vi "Teleop.vi"(10 "Match Info":T4={"Autonomous Elapsed Seconds"=0.0, "TeleOp Elapsed Seconds"=60.541, "Disabled Elapsed Seconds"=98.983, "Visited Autonomous"=FALSE, "Visited TeleOp"=TRUE, "Visited Disabled"=TRUE, "Autonomous Settings"={"Autonomous Style"=enum."Independent", "VI Refnum"=refnum}}, 11 "Call Context":T5=enum."Stop") -> ()   [LabVIEW 2016]
doc: "This VI is called for each TeleOp packet received from the DS where the robot is not disabled. It is often used to read from the joysticks and update I/O or to update setpoints for timed control loops. It should complete and return within 20 milliseconds or it may miss DS packets."
uses:
  <vilib>/Rock Robotics/WPI/DriverStation/WPI_DriverStationDerivedRobotMode.ctl
  <vilib>/Rock Robotics/WPI/DriverStation/WPI_DriverStationMatch Info.ctl
  <vilib>/Rock Robotics/WPI/Solenoid/WPI_SolenoidValue.ctl
  <vilib>/Rock Robotics/WPI/Utilities/WPI_GetSetVariantRefNum.vi
  <vilib>/Rock Robotics/Network Tables/NT Write Boolean Array.vi
  <vilib>/Rock Robotics/Network Tables/NT Write Numeric Array.vi
  <vilib>/Rock Robotics/Network Tables/NT Read Boolean.vi
  <vilib>/Rock Robotics/Network Tables/NT Read Number.vi
  <vilib>/Rock Robotics/WPI/Solenoid/WPI_SolenoidSetEnum.vi
  <vilib>/addons/control/pid/pid.llb/PID (DBL).vi
  <vilib>/Rock Robotics/WPI/RobotDrive/WPI_RobotDriveMecanumDrive_Cartesian.vi
  <vilib>/Rock Robotics/Network Tables/NT Write Number.vi
  <vilib>/addons/control/pid/NI_PID_pid.lvlib
panel:
  in  "climberpower":dbl(slide)=0.3 scale=0.0..1.0
  in  "deadband thing":dbl=0.13
  in  "Strafe":dbl(slide)=0.5 caption="Strafe Scale" scale=0.0..1.0
  in  "Deadband":dbl(slide) scale=-1.0..1.0
  out "useless data point LOL":dbl=-122.49
  out "derivative time (Td, min)":dbl
  out "integral time (Ti, min)":dbl=0.01
  out "proportional gain (Kc)":dbl=1.0
  out "Yaw":dbl=-122.49
  out "Data":T1(graph)={"setpoint"=0.0, "Yaw"=-122.49, "dt out (s)"=0.02300000109244138}
  in  "setpoint":dbl(slide) scale=-50.0..50.0
  in  "PID gains":T2={"proportional gain (Kc)"=1.0, "integral time (Ti, min)"=0.01, "derivative time (Td, min)"=0.0} {"derivative time (Td, min)" scale=0.0..0.05; "integral time (Ti, min)" scale=0.0..0.00243; "proportional gain (Kc)" scale=0.0..0.284195}
  out "YRPHfH":T3={"Yaw"=-122.49, "Roll"=8.03, "Pitch"=-3.82, "Heading"=0.0, "Fused Heading"=237.5}
  out "Sample Slider 0":dbl(slide) scale=0.0..5.0
  out "Sample Boolean 1":bool
  out "Sample Boolean 0":bool
  # "z check should be about 3-5 (in degrees)"
  # "do not mess with PID gain values"
  # "do not mess with PID gain values"
  # "do not mess with PID gain values"
  # "do not mess with PID gain values"
  # "do not mess with PID gain values"
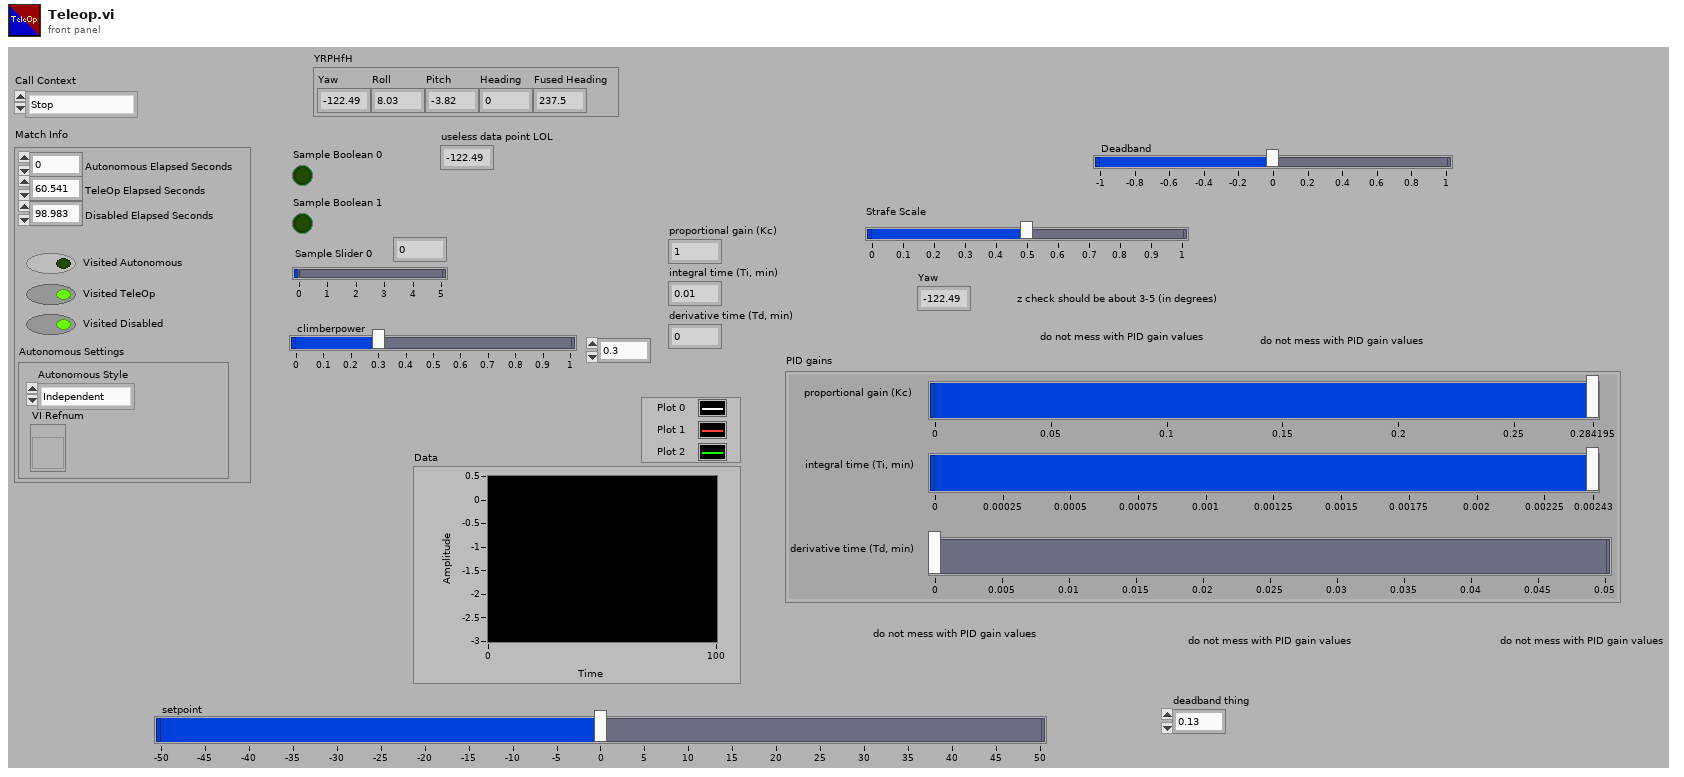
[diagram p1: front panel]
types:
  T1 = cluster{"setpoint":dbl, "Yaw":dbl, "dt out (s)":dbl}
  T2 = cluster{"proportional gain (Kc)":dbl, "integral time (Ti, min)":dbl, "derivative time (Td, min)":dbl}
  T3 = cluster{"Yaw":dbl, "Roll":dbl, "Pitch":dbl, "Heading":dbl, "Fused Heading":dbl}
  T4 = typedef "WPI_DriverStationMatch Info.ctl" = cluster{"Autonomous Elapsed Seconds":dbl, "TeleOp Elapsed Seconds":dbl, "Disabled Elapsed Seconds":dbl, "Visited Autonomous":bool, "Visited TeleOp":bool, "Visited Disabled":bool, "Autonomous Settings":cluster{"Autonomous Style":enum16{"Iterative", "Independent"}, "VI Refnum":refnum<vi>}}
  T5 = typedef "WPI_DriverStationDerivedRobotMode.ctl" = enum16{"Init", "Execute", "Stop"}
  T6 = typedef "WPI_SolenoidValue.ctl" = enum16{"Off", "On", "Forward", "Reverse"}
  T7 = typedef "WPI_JoystickDevRef.ctl" = cluster{"Device":T8}
  T8 = typedef "WPI_JoystickDeviceEnum.ctl" = enum16{"USB 0", "USB 1", "USB 2", "USB 3", "USB 4", "USB 5"}
  T9 = typedef "WPI_MotorControlDeviceRef.ctl" = cluster{"DeviceStatus":errorcluster, "Type":T10, "PWM":cluster{"PWM Channel":T11, "DeadBand":T12}, "CAN":cluster{"Device Number":u8, "SetOutput VI Ref":variant, "GetOutput VI Ref":variant, "Enable VI Ref":variant, "Disable VI Ref":variant, "Data":variant}, "Invert":bool}
  T10 = typedef "WPI_MotorControlType.ctl" = enum16{"PWM", "CAN"}
  T11 = typedef "FPGA_DIOPWMChannel.ctl" = enum8{"PWM 0", "PWM 1", "PWM 2", "PWM 3", "PWM 4", "PWM 5", "PWM 6", "PWM 7", "PWM 8", "PWM 9", "PWM MXP 0", "PWM MXP 1", "PWM MXP 2", "PWM MXP 3", "PWM MXP 4", "PWM MXP 5", "PWM MXP 6", "PWM MXP 7", "PWM MXP 8", "PWM MXP 9", "Invalid"}
  T12 = typedef "WPI_PWMDeadband.ctl" = cluster{"Name":string, "maxPositivePwm":i32, "minPositivePwm":i32, "centerPwm":i32, "maxNegativePwm":i32, "minNegativePwm":i32, "angularRange":u16}
  T13 = typedef "WPI_SolenoidDevRef.ctl" = cluster{"DevStatus":errorcluster, "Pneumatics Control Module":u8, "Forward Solenoid Channel":T14, "Reverse Solenoid Channel":T14}
  T14 = typedef "WPI_SolenoidChannel.ctl" = enum8{"Solenoid 0", "Solenoid 1", "Solenoid 2", "Solenoid 3", "Solenoid 4", "Solenoid 5", "Solenoid 6", "Solenoid 7", "Invalid"}
  T15 = typedef "WPI_RobotDriveDevRef.ctl" = cluster{"DevStatus":errorcluster, "Motors[]":T9[], "Square Inputs":bool, "Max Output":dbl}
  T16 = typedef "WPI_CompressorDevRef.ctl" = cluster{"DevStatus":errorcluster, "Pneumatics Control Module":u8}
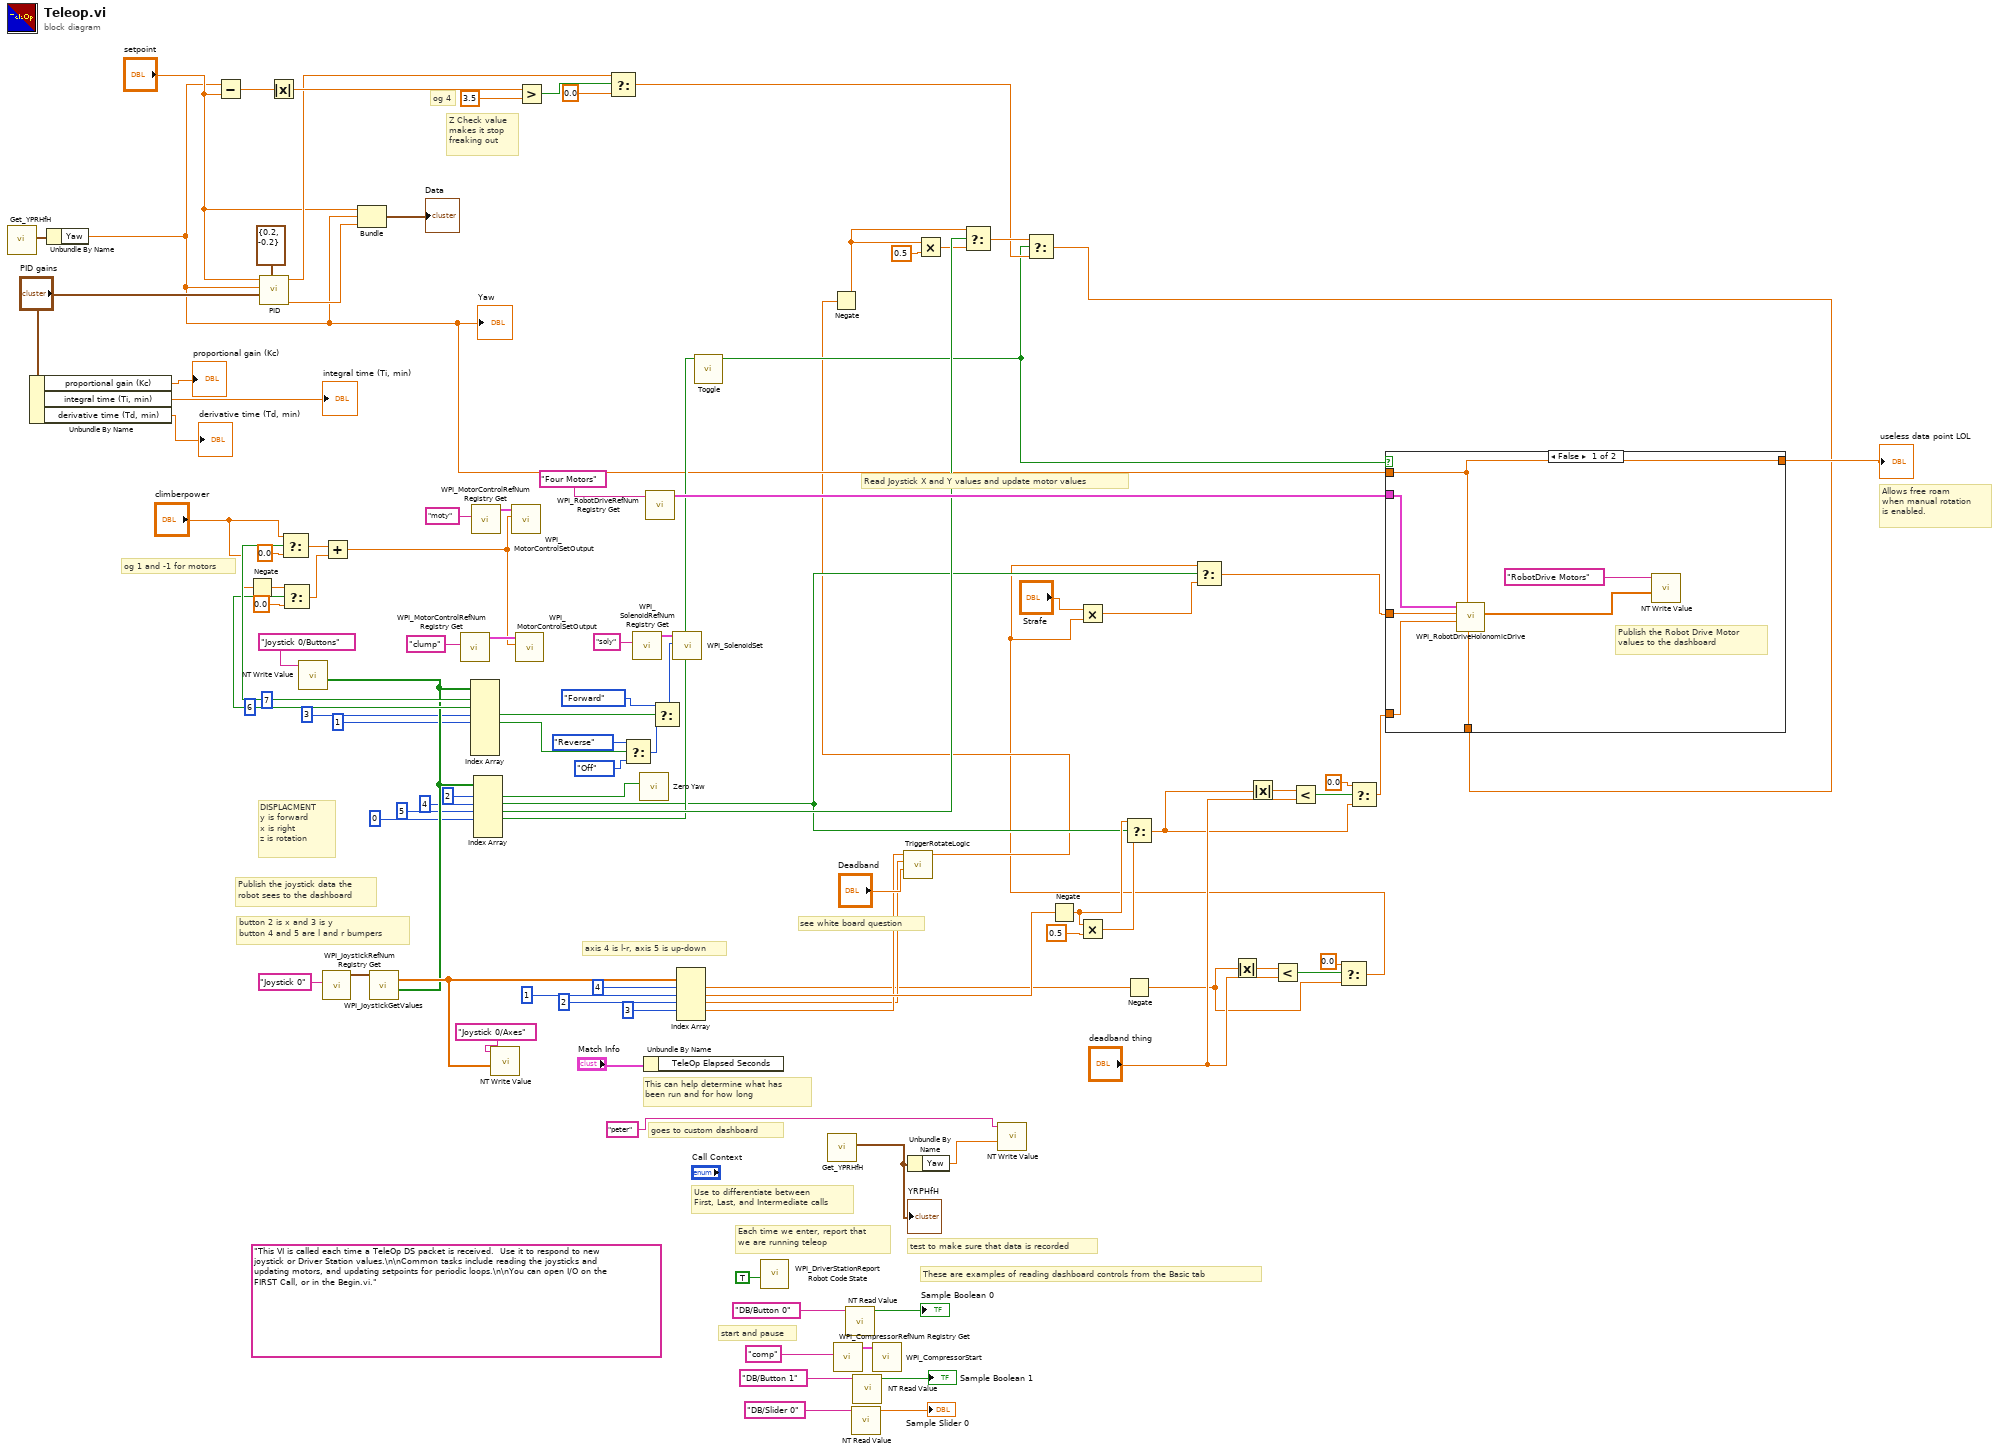
[diagram p0: block diagram]
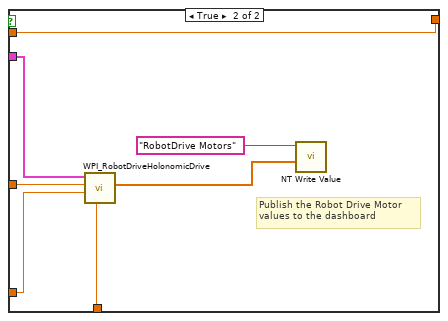
[diagram p2: hidden frame]
diagram:
  (unwired) "This VI is called each time a TeleOp DS packet is received.  Use it to respond to new joystick or Driver Station values.\n\nCommon tasks include reading the joysticks and updating motors, and updating setpoints for periodic loops.\n\nYou can open I/O on the FIRST Call, or in the Begin.vi."
  # "see white board question"
  # "axis 4 is l-r, axis 5 is up-down"
  # "og 1 and -1 for motors"
  # "og 4"
  # "Allows free roam\nwhen manual rotation\nis enabled."
  # "Z Check value\nmakes it stop\nfreaking out"
  # "start and pause"
  # "goes to custom dashboard"
  # "button 2 is x and 3 is y\nbutton 4 and 5 are l and r bumpers"
  # "DISPLACMENT\ny is forward\nx is right\nz is rotation"
  # "test to make sure that data is recorded"
  # "These are examples of reading dashboard controls from the Basic tab"
  # "Publish the joystick data the\nrobot sees to the dashboard"
  # "Each time we enter, report that\nwe are running teleop"
  # "Use to differentiate between\nFirst, Last, and Intermediate calls"
  # "This can help determine what has\nbeen run and for how long"
  # "Read Joystick X and Y values and update motor values"
  n1 = call <vilib>:"Get_YPRHfH.vi"() -> ("YRPHfH"=w49:T3)  [unwired: 11 in]
  n2 = Unbundle By Name("PID gains") -> ("proportional gain (Kc)"=→"proportional gain (Kc)":dbl, "integral time (Ti, min)"=→"integral time (Ti, min)":dbl, "derivative time (Td, min)"=→"derivative time (Td, min)":dbl)
  n3 = Unbundle By Name(w49) -> ("Yaw"=w15:dbl)
  "Yaw" <- w15
  n4 = Subtract(x=w15, y="setpoint") -> (x-y=w53:dbl)
  n5 = Negate(x="climberpower") -> (-x=w1:dbl)
  n6 = call-poly <vilib>:"PID.vi"("output range"=cluster{"output high":dbl, "output low":dbl} {"output high"=0.2, "output low"=-0.2}, "PID gains"="PID gains", "process variable"=w15, "setpoint"="setpoint") -> ("dt out (s)"=w46:dbl, "output"=w45:dbl)  [unwired: 6 in]
  n7 = Absolute Value(x=w53) -> (abs(x)=w54:dbl)
  n8 = call <vilib>:"WPI_JoystickRefNum Registry Get.vi"("refnum name"="Joystick 0") -> ("JoystickDevRef"=w102:T7)  [unwired: 1 in, 9 out]
  n9 = Bundle("setpoint"="setpoint", "Yaw"=w15, "dt out (s)"=w46) -> (→"Data":T1)  [unwired: 1 in]
  n10 = call <vilib>:"WPI_JoystickGetValues.vi"("JoystickDevRef"=w102) -> ("Buttons"=w70:bool[], "Axes"=w99:dbl[])  [unwired: 6 in, 3 out]
  n11 = call-poly <vilib>:"NT Write Value.vi"("Boolean Array"=w70, "Name"="Joystick 0/Buttons") -> ()  [unwired: 9 in, 1 out]
  n12 = call <vilib>:"WPI_MotorControlRefNum Registry Get.vi"("refnum name"="clump") -> ("MotorControlDevRef"=w62:T9)  [unwired: 9 in, 1 out]
  n13 = Index Array(array=w70, index #1=7 ("index"), index #2=6 ("index"), index #3=3 ("index"), index #4=1 ("index")) -> (element #1=w87:bool, element #2=w86:bool, element #3=w23:bool, element #4=w21:bool)  [unwired: 4 in, 4 out]
  n14 = Select(t="climberpower", s=w87, f=0.0) -> (s? t:f=w83:dbl)
  n15 = Select(t=w1, s=w86, f=0.0) -> (s? t:f=w82:dbl)
  n16 = Add(x=w83, y=w82) -> (x+y=w61:dbl)
  n17 = call <vilib>:"WPI_MotorControlRefNum Registry Get.vi"("refnum name"="moty") -> ("MotorControlDevRef"=w88:T9)  [unwired: 9 in, 1 out]
  n18 = Index Array(array=w70, index #1=2 ("index"), index #2=4 ("index"), index #3=5 ("index"), index #4=0 ("index")) -> (element #1=w18:bool, element #2=w9:bool, element #3=w66:bool, element #4=w41:bool)  [unwired: 2 in, 2 out]
  n19 = call-poly <vilib>:"NT Write Value.vi"("Numeric Array"=w99, "Name"="Joystick 0/Axes") -> ()  [unwired: 9 in, 1 out]
  n20 = call <vilib>:"WPI_MotorControlSetOutput.vi"("Output"=w61, "MotorControlDevRef"=w88) -> ()  [unwired: 7 in, 3 out]
  n21 = call <vilib>:"WPI_MotorControlSetOutput.vi"("Output"=w61, "MotorControlDevRef"=w62) -> ()  [unwired: 7 in, 3 out]
  n22 = Greater?(x=w54, y=3.5) -> (0:w14:bool)
  n23 = Select(t=w45, s=w14, f=0.0) -> (s? t:f=w47:dbl)
  n24 = Select(t=WPI_SolenoidValue."Reverse" ("Value"), s=w21, f=WPI_SolenoidValue."Off" ("Value")) -> (s? t:f=w24:T6)
  n25 = call <vilib>:"WPI_SolenoidRefNum Registry Get.vi"("refnum name"="soly") -> ("SolenoidDevRef"=w80:T13)  [unwired: 9 in, 1 out]
  n26 = call <vilib>:"Zero Yaw.vi"("Zero"=w18) -> ()  [unwired: 11 in]
  n27 = Unbundle By Name("Match Info") -> ()  [unwired: 1 out]
  n28 = call <vilib>:"WPI_RobotDriveRefNum Registry Get.vi"("refnum name"="Four Motors") -> ("RobotDriveDevRef"=w104:T15)  [unwired: 1 in, 9 out]
  n29 = Select(t=WPI_SolenoidValue."Forward" ("Value"), s=w23, f=w24) -> (s? t:f=w79:T6)
  n30 = call-poly <vilib>:"WPI_SolenoidSet.vi"("Value"=w79, "SolenoidDevRef"=w80) -> ()  [unwired: 8 in, 2 out]
  n31 = Index Array(array=w99, index #1=4 ("index"), index #2=1 ("index"), index #3=2 ("index"), index #4=3 ("index")) -> (element #1=w27:dbl, element #2=w58:dbl, element #3=w34:dbl, element #4=w35:dbl)  [unwired: 1 in, 1 out]
  n32 = call "Toggle.vi"("Button Input"=w41) -> ("Toggle Output"=w13:bool)  [unwired: 9 in, 1 out]
  n33 = call <vilib>:"WPI_DriverStationReport Robot Code State.vi"("TeleOp"=TRUE ("Autonomous")) -> ()  [unwired: 10 in, 1 out]
  n34 = call <vilib>:"Get_YPRHfH.vi"() -> ("YRPHfH"=w19:T3)  [unwired: 11 in]
  "YRPHfH" <- w19
  n35 = call <vilib>:"WPI_CompressorRefNum Registry Get.vi"("refnum name"="comp") -> ("CompressorDevRef"=w81:T16)  [unwired: 9 in, 1 out]
  n36 = call-poly <vilib>:"NT Read Value.vi"("Name"="DB/Button 0" ("refnum name")) -> ("Boolean"=→"Sample Boolean 0":bool)  [unwired: 9 in, 1 out]
  n37 = call-poly <vilib>:"NT Read Value.vi"("Name"="DB/Slider 0" ("refnum name")) -> ("Numeric"=→"Sample Slider 0":dbl)  [unwired: 9 in, 1 out]
  n38 = call-poly <vilib>:"NT Read Value.vi"("Name"="DB/Button 1" ("refnum name")) -> ("Boolean"=→"Sample Boolean 1":bool)  [unwired: 9 in, 1 out]
  n39 = call <vilib>:"WPI_CompressorStart.vi"("CompressorDevRef"=w81) -> ()  [unwired: 9 in, 2 out]
  n40 = call "TriggerRotateLogic.vi"("Deadband"="Deadband", "Right Trigger"=w34, "Left Trigger"=w35) -> ("Output"=w6:dbl)  [unwired: 8 in]
  n41 = Negate(x=w6) -> (-x=w3:dbl)
  n42 = Unbundle By Name(w19) -> ("Yaw"=w72:dbl)
  n43 = Multiply(x=w3, y=0.5) -> (x*y=w65:dbl)
  n44 = Select(t=w3, s=w66, f=w65) -> (s? t:f=w48:dbl)
  n45 = call-poly <vilib>:"NT Write Value.vi"("Numeric"=w72, "Name"="peter") -> ()  [unwired: 9 in, 1 out]
  n46 = Select(t=w48, s=w13, f=w47) -> (s? t:f=w7:dbl)
  n47 = Negate(x=w58) -> (-x=w37:dbl)
  n48 = Multiply(x=w37, y=0.5) -> (x*y=w57:dbl)
  n49 = Select(t=w37, s=w9, f=w57) -> (s? t:f=w8:dbl)
  n50 = Negate(x=w27) -> (-x=w4:dbl)
  n51 = Absolute Value(x=w4) -> (abs(x)=w25:dbl)
  n52 = Absolute Value(x=w8) -> (abs(x)=w30:dbl)
  n53 = Less?(x=w25, y="deadband thing") -> (x < y?=w28:bool)
  n54 = Less?(x=w30, y="deadband thing") -> (x < y?=w33:bool)
  n55 = Select(t=0.0, s=w28, f=w4) -> (s? t:f=w5:dbl)
  n56 = Multiply(x="Strafe", y=w5) -> (x*y=w11:dbl)
  n57 = Select(t=w5, s=w9, f=w11) -> (s? t:f=w10:dbl)
  n58 = Select(t=0.0, s=w33, f=w8) -> (s? t:f=w31:dbl)
  n59 = case shown="False" w13 {
    tunnel: w104 -> [w109 w120]
    tunnel: w31 -> [w111 w117]
    tunnel: w10 -> [w110 w116]
    tunnel: w15 -> [w108 w115]
    tunnel: [w108 w115] -> w39
    tunnel: w7 -> [w107 w114]
    frame False {
      # "Publish the Robot Drive Motor\nvalues to the dashboard"
      n60 = call-poly <vilib>:"WPI_RobotDriveHolonomicDrive.vi"("Rotation"=w107, "Gyro Angle"=w108, "Y"=w111, "X"=w110, "RobotDriveDevRef"=w109) -> ("Motor Values"=w112:dbl[])  [unwired: 4 in, 2 out]
      n61 = call-poly <vilib>:"NT Write Value.vi"("Numeric Array"=w112, "Name"="RobotDrive Motors") -> ()  [unwired: 9 in, 1 out]
    }
    frame True {
      # "Publish the Robot Drive Motor\nvalues to the dashboard"
      n62 = call-poly <vilib>:"WPI_RobotDriveHolonomicDrive.vi"("Rotation"=w114, "Y"=w117, "X"=w116, "RobotDriveDevRef"=w120) -> ("Motor Values"=w118:dbl[])  [unwired: 5 in, 2 out]
      n63 = call-poly <vilib>:"NT Write Value.vi"("Numeric Array"=w118, "Name"="RobotDrive Motors") -> ()  [unwired: 9 in, 1 out]
    }
  }
  "useless data point LOL" <- w39
